vi "Robot Global Data.vi"() -> ()   [LabVIEW 2018]
doc: "This global VI can contain as many global variables as you need. Place a control on the panel, give it a good name. To read or write to it from a VI, drag the icon to the diagram of that VI. You can also drag from the project. Click on the node to change which global you access. You shouldn't have multiple locations writing to a global or it will cause a race-condition."
uses:
  <vilib>/Rock Robotics/WPI/Camera/WPI_CameraImageSize.ctl
  <vilib>/Rock Robotics/WPI/DriverStation/WPI_DriverStationRobotMode2.ctl
panel:
  out "Auto Complete":bool
  in  "Elevator Setpoint":dbl
  in  "Wrist Direction":enum16{"Wrist Front", "Wrist Back"}(ring)
  in  "Robot State":T1(ring)
  in  "Robot Mode":T2
  in  "image size":T3=enum."320x240"
  in  "Enable Vision":bool
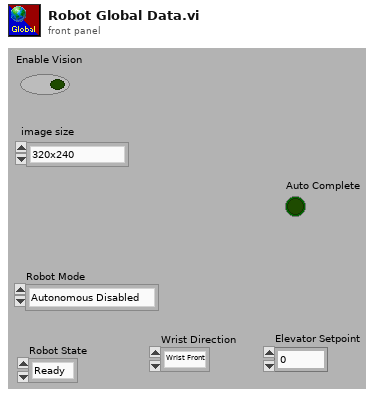
[diagram p1: front panel]
types:
  T1 = enum16{"Ready", "Stow", "Intake Hatch", "Intake Cargo", "Floor Cargo", "Go To Hatch", "Go To Cargo", "Score Hatch - Extend", "Score Hatch - Claw Closed", "Score Hatch - Retract", "Score Cargo - Extend", "Score Cargo - Claw Open", "Score Cargo - Retract"}
  T2 = typedef "WPI_DriverStationRobotMode2.ctl" = enum16{"Autonomous Disabled", "Autonomous Enabled", "Teleop Disabled", "Teleop Enabled", "Disconnected", "Finish", "Test Disabled", "Test Enabled", "Emergency Stopped"}
  T3 = typedef "WPI_CameraImageSize.ctl" = enum16{"640x480", "320x240", "160x120", "Custom"}
diagram:
